vi "Format CSV.vi"(8 "error in (no error)":errorcluster, 9 "delimiter":string=",", 10 "CSV File Input":path, 11 "Original CSV Format":enum16{"OGnE", "WAN-OGE"}(ring)) -> (0 "error out":errorcluster, 1 "Parcel Length":i32[](array[numeric]), 3 "All Terminal Data":T1[](array[typedef]))   [LabVIEW 2017] (continued)
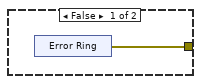
[diagram p3: hidden frame]
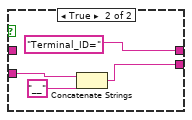
[diagram p5: hidden frame]
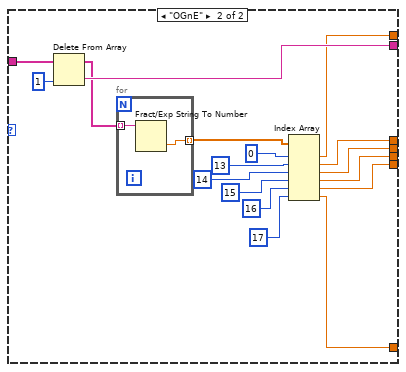
[diagram p6: hidden frame]
      n69 = Index Array(array=w190, index (row)=w206) -> (element=w191:string[])  [unwired: 1 in]
      n70 = Delete From Array(array=w191, index=0 ("disabled index (col)")) -> (deleted portion=w188:string, array with subset deleted=w187:string[])  [unwired: 1 in]
      n71 = case shown="\"WAN-OGE\", Default" w204 {
        tunnel: w187 -> [w212 w244]
        tunnel: ["" ("String") w243] -> w203
        tunnel: [w219 w229] -> w202
        tunnel: [w217 w240] -> w201
        tunnel: [w216 w239] -> w200
        tunnel: [w215 w238] -> w199
        tunnel: [w214 w231] -> w197
        tunnel: [w213 w237] -> w196
        frame "WAN-OGE", Default {
          n72 = Delete From Array(array=w212) -> (array with subset deleted=w211:string[])  [unwired: 2 in, 1 out]
          n73 = for {
            tunnel: [w227] -> w225 mode=indexing
            tunnel: w211 -> [w228] mode=indexing
            n74 = Fract/Exp String To Number(string=w228) -> (number=w227:dbl)  [unwired: 3 in, 1 out]
          }
          n75 = Index Array(array=w225, index #1=0 ("index"), index #2=4 ("index"), index #3=5 ("index"), index #4=2 ("index"), index #5=3 ("index"), index #6=6 ("index")) -> (element #1=w219:dbl, element #2=w217:dbl, element #3=w216:dbl, element #4=w215:dbl, element #5=w214:dbl, element #6=w213:dbl)
        }
        frame "OGnE" {
          n76 = Delete From Array(array=w244, index=1) -> (deleted portion=w243:string, array with subset deleted=w242:string[])  [unwired: 1 in]
          n77 = for {
            tunnel: [w246] -> w241 mode=indexing
            tunnel: w242 -> [w247] mode=indexing
            n78 = Fract/Exp String To Number(string=w247) -> (number=w246:dbl)  [unwired: 3 in, 1 out]
          }
          n79 = Index Array(array=w241, index #1=0 ("index"), index #2=13 ("index"), index #3=14 ("index"), index #4=15 ("index"), index #5=16 ("index"), index #6=17 ("index")) -> (element #1=w229:dbl, element #2=w240:dbl, element #3=w239:dbl, element #4=w238:dbl, element #5=w231:dbl, element #6=w237:dbl)
        }
      }
      n80 = expression code="(x/180.0)*pi" ("degrees to radians")(w197) -> (w198:dbl)
      n81 = expression code="(x/180.0)*pi" ("degrees to radians")(w200) -> (w205:dbl)
      n82 = Polar To Complex(1:w205, 2:w201) -> (0:w195:cdb)
      n83 = Polar To Complex(1:w198, 2:w199) -> (0:w194:cdb)
      n84 = Complex Conjugate(1:w194) -> (0:w193:cdb)
      n85 = Multiply(x=w195, y=w193) -> (x*y=w192:cdb)
    }
    n86 = Complex To Re/Im(x + iy=w171) -> (x=w163:dbl[], y=w164:dbl[])
    n87 = Complex To Re/Im(x + iy=w170) -> (x=w165:dbl[], y=w166:dbl[])
    n88 = Complex To Re/Im(x + iy=w169) -> (x=w167:dbl[], y=w168:dbl[])
    n89 = Current VI's Path() -> (path=w159:path)
    n90 = Number To Decimal String(number=w130) -> (decimal integer string=w129:string)  [unwired: 1 in]
    n91 = Equal?(x=w132, y="") -> (x = y?=w155:bool)
    n92 = case shown="False" w155 {
      tunnel: ["_" ("string") w184] -> w136
      tunnel: [w182 "Terminal_ID=" ("string")] -> w137
      tunnel: w132 -> [w182 _]
      tunnel: w129 -> [_ w186]
      frame False {
      }
      frame True {
        n93 = Concatenate Strings "Concatenate Strings"(w186, "__" ("string")) -> (w184:string)
      }
    }
    n94 = Number To Fractional String(number=w163) -> (F-format string=w150:string[])  [unwired: 3 in]
    n95 = Strip Path(path=w159) -> (stripped path=w160:path)  [unwired: 1 out]
    n96 = Number To Fractional String(number=w164) -> (F-format string=w149:string[])  [unwired: 3 in]
    n97 = Number To Fractional String(number=w165) -> (F-format string=w148:string[])  [unwired: 3 in]
    n98 = Number To Fractional String(number=w166) -> (F-format string=w147:string[])  [unwired: 3 in]
    n99 = Number To Fractional String(number=w167) -> (F-format string=w146:string[])  [unwired: 3 in]
    n100 = Number To Fractional String(number=w162, precision (6)=i16 5) -> (F-format string=w144:string[])  [unwired: 2 in]
    n101 = Index Array(array=w151, index=0) -> (element=w131:string)
    n102 = Number To Fractional String(number=w168) -> (F-format string=w145:string[])  [unwired: 3 in]
    n103 = Path To String(path=w160) -> (string=w153:string)
    n104 = Search and Replace String(replace all?=TRUE ("replace all? (F)"), input string=w131, search string=":", replace string="_" ("replace string (\"\")")) -> (result string=w122:string)  [unwired: 4 in, 3 out]
    n105 = call <vilib>:"Space Constant.vi"() -> ("String"=w121:string)
    n106 = Build Array(w151, w150, w149, w148, w147, w146, w145, w144) -> (w143:string[][])
    n107 = Search and Replace String(replace all?=TRUE ("replace all? (F)"), input string=w122, search string=w121, replace string="__" ("replace string (\"\")")) -> (result string=w123:string)  [unwired: 4 in, 3 out]
    n108 = local read "delimiter"() -> (w175:string)
    n109 = Transpose 2D Array(2D array=w143) -> (transposed array=w142:string[][])
    n110 = Build Array (concatenate)(string[] ["Timestamps", "Real Voltage", "Imag. Voltage", "Real Current", "Imag. Current", "Real Power", "Apparent Power", "Frequency"] ("Array"), w142) -> (w140:string[][])
    n111 = Concatenate Strings "Concatenate Strings"(w153, "\\CSV_Files\\" ("string"), w137, w136, w123, ".csv" ("string")) -> (w161:string)
    n112 = String To Path(string=w161) -> (path=w154:path)
    n113 = call-poly <vilib>:"Write Delimited Spreadsheet.vi"("file path (dialog if empty)"=w154, "2D data"=w140, "append to file? (new file:F)"=FALSE, "error in (no error)"=w180, "delimiter (\\t)"=w175) -> ("new file path (Not A Path if cancelled)"=w174:path, "error out"=w179:errorcluster)  [unwired: 9 in]
    n114 = Bundle By Name(cluster=T3 {"Terminal Data"=path "", "Terminal ID"=0.0, "Terminal Name"=""} ("Cluster"), "Terminal ID"=w130, "Terminal Name"=w132, "Terminal Data"=w174) -> (w173:T3)
  }
  "error out" <- w41
  "All Terminal Data" <- w28
